vi "Pause.vi"(8 "error in (no error)":errorcluster, 11 "Sonicator Module State Cluster":T1={"State"=enum."Idle", "Start Time"=timestamp(0 s since 1904-01-01), "Current Time"=timestamp(0 s since 1904-01-01), "Sonicator Module Config"={"GUID"="", "Drop Coords"={"Horizontal"=0, "Vertical"=0}, "Process Name"="", "Queue Name"="", "Settings"={"Cycle Period"=500.0, "Sonicator Type"="", "SS P100 Settings"={"VISA resource name"="", "Simulated?"=FALSE}, "Setpoint (µm)"=0.0, "Cutoff (µm)"=0.0}, "Load Count"=0}, "Output Error"=FALSE, "Log Started"=FALSE, "First Iteration"=FALSE, "Data"={"Sonicator Amp Value"=0.0, "Sonicator Power Value"=0.0}, "Sonicator On?"=enum."Off"}) -> (0 "error out":errorcluster, 3 "Sonicator Module State Cluster":T1={"State"=enum."Idle", "Start Time"=timestamp(0 s since 1904-01-01), "Current Time"=timestamp(0 s since 1904-01-01), "Sonicator Module Config"={"GUID"="", "Drop Coords"={"Horizontal"=0, "Vertical"=0}, "Process Name"="", "Queue Name"="", "Settings"={"Cycle Period"=500.0, "Sonicator Type"="", "SS P100 Settings"={"VISA resource name"="", "Simulated?"=FALSE}, "Setpoint (µm)"=0.0, "Cutoff (µm)"=0.0}, "Load Count"=0}, "Output Error"=FALSE, "Log Started"=FALSE, "First Iteration"=FALSE, "Data"={"Sonicator Amp Value"=0.0, "Sonicator Power Value"=0.0}, "Sonicator On?"=enum."Off"})   [LabVIEW 2018, in "Sonicator Module.lvlib" / "Sonicator Module Engine.lvlib"]
uses:
  Sonicator Module Engine.lvlib
  Feed Module/Controls/Sonicator Module State Cluster.ctl
  Pump Module Folder/Measure Instrument/State Enum.ctl
  Feed Module/Controls/Sonicator Module Config Cluster.ctl
  <vilib>/Utility/miscctls.llb/LVPoint32TypeDef.ctl
  Feed Module/Controls/Sonicator Module Settings Cluster.ctl
  Sonic Systems P100/Sonic Systems P100 Settings.ctl
  Tag VIs/Tag FGV Operation Enum.ctl
  Shared Variables/Dynamic Shared Variables.lvlib
  Sonic Systems P100/Sonic Systems P100.lvlib
  Pump Module Folder/Measure Instrument/Pump Module Engine.lvlib
  Sonicator Module.lvlib
panel:
  # "Sonicator Settings"
  # "Sonicator Settings"
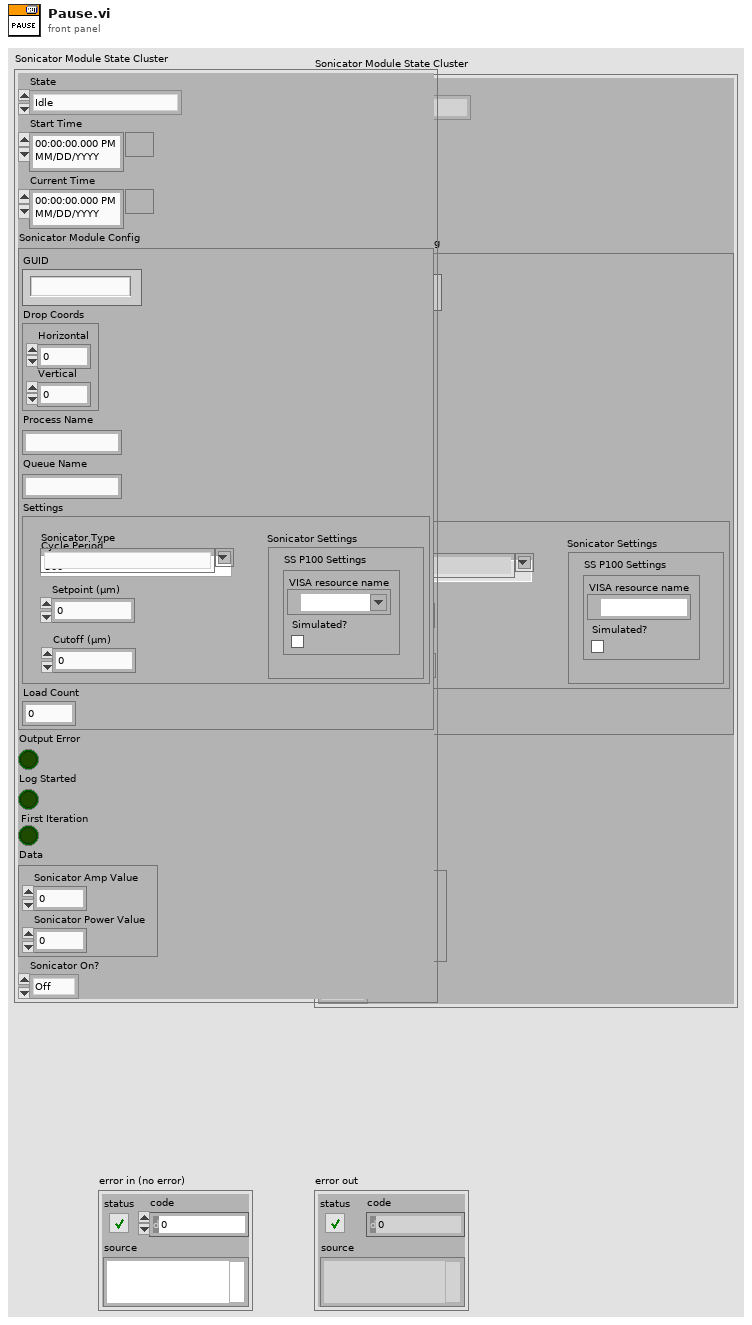
[diagram p1: front panel]
types:
  T1 = typedef "Sonicator Module.lvlib/Sonicator Module State Cluster.ctl" = cluster{"State":T2, "Start Time":timestamp, "Current Time":timestamp, "Sonicator Module Config":T3, "Output Error":bool, "Log Started":bool, "First Iteration":bool, "Data":cluster{"Sonicator Amp Value":dbl, "Sonicator Power Value":dbl}, "Sonicator On?":enum16{"Off", "On", "Not Initialized"}}
  T2 = typedef "Pump Module.lvlib/Pump Module Engine.lvlib/State Enum.ctl" = enum16{"Measuring", "Idle", "Paused"}
  T3 = typedef "Sonicator Module.lvlib/Sonicator Module Config Cluster.ctl" = cluster{"GUID":string, "Drop Coords":T4, "Process Name":string, "Queue Name":string, "Settings":T5, "Load Count":i32}
  T4 = typedef "LVPoint32TypeDef.ctl" = cluster{"Horizontal":i32, "Vertical":i32}
  T5 = typedef "Sonicator Module.lvlib/Sonicator Module Settings Cluster.ctl" = cluster{"Cycle Period":dbl, "Sonicator Type":string, "SS P100 Settings":T6, "Setpoint (µm)":dbl, "Cutoff (µm)":dbl}
  T6 = typedef "Sonic Systems P100.lvlib/Sonic Systems P100 Settings.ctl" = cluster{"VISA resource name":refnum<visa-resource-name>, "Simulated?":bool}
  T7 = cluster{"Amplitude Tag":string, "Power Tag":string, "Output Device Tag":string}
  T8 = typedef "Tag FGV Operation Enum.ctl" = enum16{"Init", "Set Notification Queue", "Create Tag", "Commit", "Write Tag (Numeric)", "Write Tag (Boolean)", "Read All Tags", "Read One Tag", "Delete Tag Category", "Set Alarm Parameters (Numeric)", "Set Alarm Parameters (Boolean)", "Enable All Alarms", "Disable All Alarms", "Delete All Tags", "Read Alarms", "Ack Alarm", "Read Alarm Parameters (Numeric)", "Read Alarm Parameters (Boolean)"}
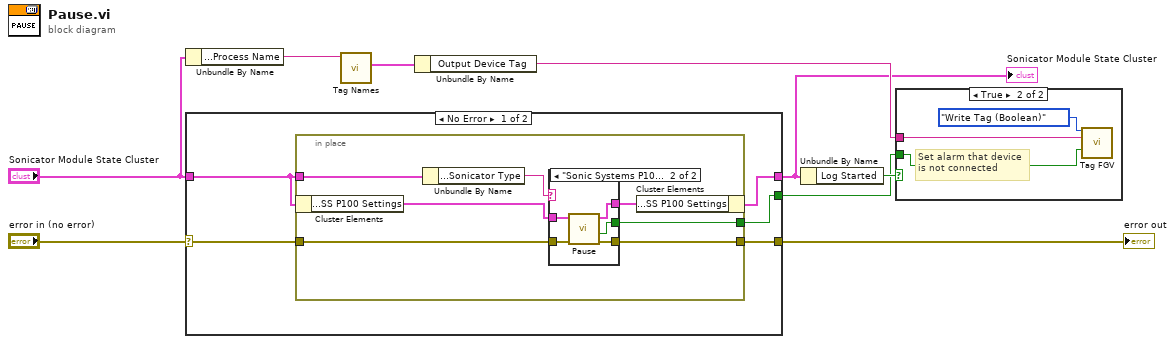
[diagram p0: block diagram]
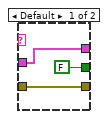
[diagram p3: hidden frame]
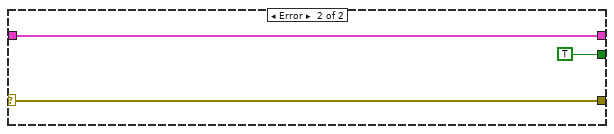
[diagram p4: hidden frame]
diagram:
  n1 = Unbundle By Name("Sonicator Module State Cluster") -> ("Sonicator Module Config.Process Name"=w1:string)
  n2 = case shown="No Error" "error in (no error)" {
    selector: "error in (no error)" -> [w13 w32]
    tunnel: [w14 w32] -> w8
    tunnel: "Sonicator Module State Cluster" -> [w10 w31]
    tunnel: [w12 w31] -> w4
    tunnel: [w11 TRUE ("Connection Error")] -> w5
    frame No Error {
      n3 = in-place {
        in-place-border: [w21] -> w14
        in-place-border: w13 -> [w20]
        in-place-border: [w17] -> w11
        in-place-border: w10 -> [w16]
        n4 = in-place-cluster #1(w10) -> ("Sonicator Module Config.Settings.SS P100 Settings"=w19:T6)
        n5 = Unbundle By Name(w16) -> ("Sonicator Module Config.Settings.Sonicator Type"=w15:string)
        n6 = case shown="\"Sonic Systems P100\"" w15 {
          tunnel: [w23 w29] -> w21
          tunnel: w20 -> [w23 w28]
          tunnel: w19 -> [w24 w27]
          tunnel: [w24 w26] -> w18
          tunnel: [FALSE ("Connection Error") w25] -> w17
          frame Default {
          }
          frame "Sonic Systems P100" {
            n7 = call "Pause.vi"("error in (no error)"=w28, "SS P100 Settings In"=w27) -> ("error out"=w29:errorcluster, "Connection Error"=w25:bool, "SS P100 Settings Out"=w26:T6)  [unwired: 7 in]
          }
        }
        n8 = in-place-cluster #1("Sonicator Module Config.Settings.SS P100 Settings"=w18) -> (w12:T1)
      }
    }
    frame Error {
    }
  }
  "error out" <- w8
  "Sonicator Module State Cluster" <- w4
  n9 = call "Tag Names.vi"("Process Name"=w1) -> ("SC Tags"=w3:T7)  [unwired: 8 in, 2 out]
  n10 = Unbundle By Name(w3) -> ("Output Device Tag"=w7:string)
  n11 = Unbundle By Name(w4) -> ("Log Started"=w6:bool)
  n12 = case shown="True" w6 {
    tunnel: w7 -> [_ w34]
    tunnel: w5 -> [_ w33]
    frame False {
    }
    frame True {
      # "Set alarm that device\nis not connected"
      n13 = call "Tag FGV.vi"("Operation"=Tag_FGV_Operation_Enum."Write Tag (Boolean)", "Tag Name"=w34, "Data"=w33) -> ()  [unwired: 5 in, 8 out]
    }
  }
